vi "Get StartStop Status.vi"(8 "error in":errorcluster, 11 "VISA resource name in":refnum<visa-resource-name>) -> (0 "error out":errorcluster, 1 "Status":bool, 3 "VISA resource name out":refnum<visa-resource-name>)   [LabVIEW 2018, in "JULABO DeviceDriver.lvlib"]
doc: "This VI returns true if the instrument is started or false if it is in Standby-Mode"
uses:
  JULABO DeviceDriver.lvlib
panel:
  out "String (output)":string
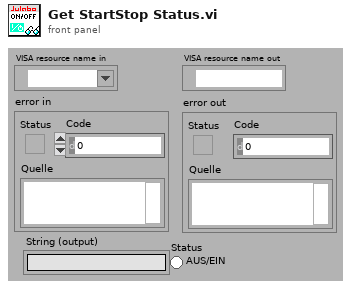
[diagram p1: front panel]
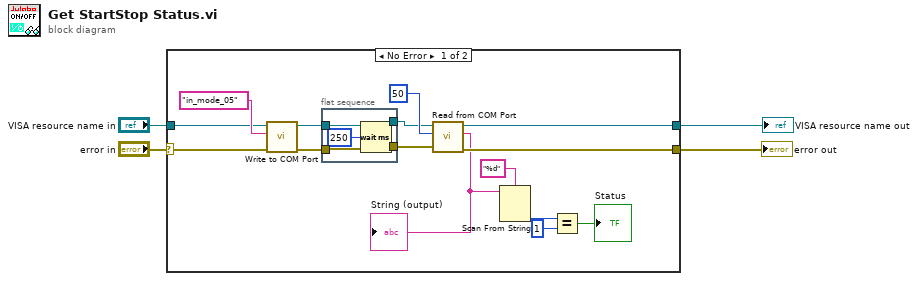
[diagram p0: block diagram]
diagram:
  n1 = case shown="No Error" "error in" {
    selector: "error in" -> [w9 w23]
    tunnel: [w18 w23] -> w4
    tunnel: [w15 w24] -> w3
    tunnel: "VISA resource name in" -> [w13 w24]
    frame No Error {
      n2 = call "Write to COM Port.vi"("error in"=w9, "Command (input)"="in_mode_05", "VISA resource name in"=w13) -> ("error out"=w5:errorcluster, "VISA resource name out"=w7:refnum<visa-resource-name>)  [unwired: 7 in]
      n3 = flat-sequence {
        tunnel: [w21] -> w8
        tunnel: w7 -> [w21]
        tunnel: [w20] -> w6
        tunnel: w5 -> [w20]
        frame #0 {
          n4 = Wait (ms)(milliseconds to wait=u32 250) -> ()  [unwired: 1 out]
        }
      }
      n5 = call "Read from COM Port.vi"("error in"=w6, "Byte to Read (-1:All)"=u32 50 ("Anzahl der Byte"), "VISA resource name in"=w8) -> ("error out"=w18:errorcluster, "String (output)"=w16:string, "VISA resource name out"=w15:refnum<visa-resource-name>)  [unwired: 5 in, 1 out]
      "String (output)" <- w16
      n6 = Scan From String(format string="%d" ("Format-String"), input string=w16) -> (output 1=w12:i32)  [unwired: 3 in, 3 out]
      n7 = Equal?(x=w12, y=1) -> (x = y?=→"Status":bool)
    }
    frame Error {
    }
  }
  "error out" <- w4
  "VISA resource name out" <- w3
